vi "Temperature Limit.vi"() -> ()   [LabVIEW 2012]
doc: "该VI可仿真温度采集，绘制温度图形，并通知用户温度是否超出范围。"
panel:
  in  "开始":bool
  in  "△t(ms)":i32(slide)=400 scale=50.0..500.0
  in  "停止":bool
  in  "上限":dbl=28.0 format="%.2f"
  out "温度":cluster{"Temperature":dbl, "High Limit":dbl}(graph)={"Temperature"=85.88749999999999, "High Limit"=80.0}
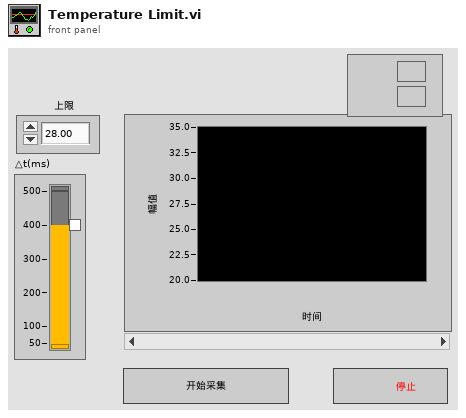
[diagram p1: front panel]
types:
  T1 = enum8{"Enabled", "Disabled", "Disabled and Grayed Out"}
  T2 = enum16{"Always On", "Always Off", "Off While Running"}
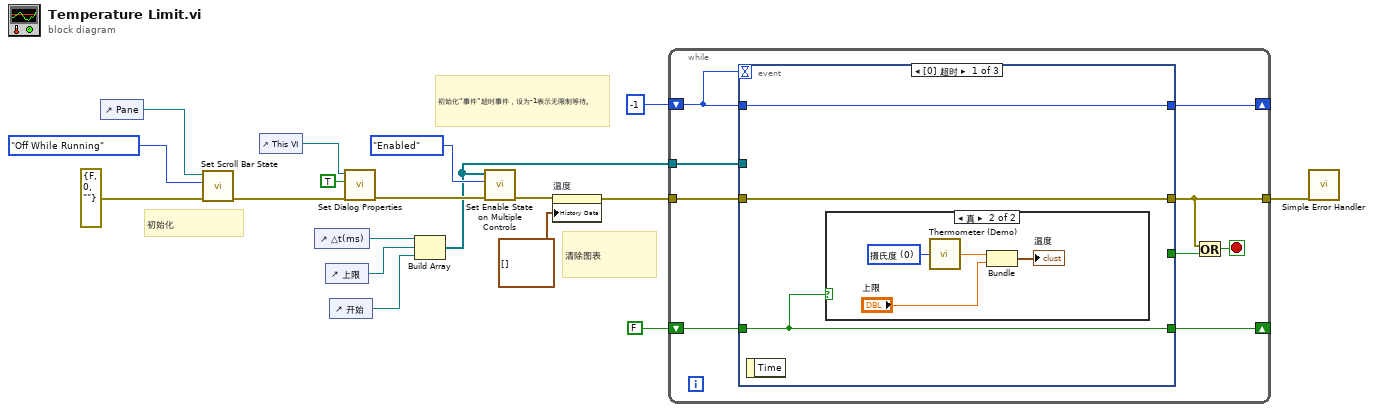
[diagram p0: block diagram]
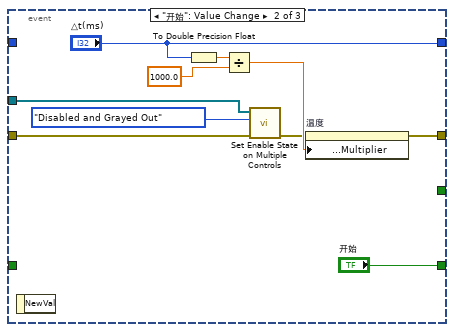
[diagram p3: hidden frame]
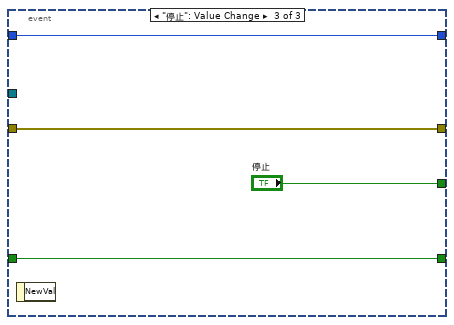
[diagram p4: hidden frame]
diagram:
  # "清除图表"
  # "初始化“事件”超时事件，设为-1表示无限制等待。"
  # "初始化"
  n1 = control-ref of="Pane"() -> (w11:refnum<vi>)
  n2 = call "Set Scroll Bar State.vi"("错误输入"=cluster{"状态":bool, "代码":i32, "源":string} {"状态"=FALSE, "代码"=0, "源"=""} ("错误输入（无错误）"), "滚动条可见（始终打开）"=T2."Off While Running", "窗格引用输入"=w11) -> ("错误输出"=w9:cluster{"状态":bool, "代码":i32, "源":string})  [unwired: 7 in, 1 out]
  n3 = control-ref of="This VI"() -> (w10:refnum<vi>)
  n4 = control-ref of="△t(ms)"() -> (w5:refnum<vi>)
  n5 = control-ref of="上限"() -> (w4:refnum<vi>)
  n6 = control-ref of="开始"() -> (w3:refnum<vi>)
  n7 = call "Set Dialog Properties.vi"("错误输入（无错误）"=w9, "启用对话框属性"=TRUE, "VI引用输入"=w10) -> ("错误输出"=w7:cluster{"状态":bool, "代码":i32, "源":string})  [unwired: 7 in, 1 out]
  n8 = Build Array ("创建数组")(w5, w4, w3) -> (w1:refnum<vi>[])
  n9 = call "Set Enable State on Multiple Controls.vi"("错误输入"=w7, "已禁用状态"=T1."Enabled", "控件"=w1) -> ("错误输出"=w6:cluster{"状态":bool, "代码":i32, "源":string})  [unwired: 8 in]
  n10 = property on="温度" class="WFChart (严格)"(error in=w6, "History Data"=cluster{"温度":dbl, "高限制":dbl}[] [] ("历史数据")) -> (error out=w17:errorcluster)  [unwired: 1 in, 1 out]
  n11 = while {
    tunnel: w17 -> [w27]
    tunnel: [w25] -> w15
    shift-right: [w23] -> _
    shift-left: FALSE ("开始") -> [w22]
    shift-right: [w21] -> _
    shift-left: -1 ("△t(ms)") -> [w20]
    tunnel: w1 -> [w19]
    stop <- w26 stop-if-true
    n12 = event shown="[0] 超时" {
      selector: _ -> [_ _ _]
      dyn-events: _ -> [_ _ _]
      timeout: w20 -> [_ _ _]
      tunnel: [_ _ "停止"] -> w24
      tunnel: w27 -> [w30 w37 w47]
      tunnel: [w30 w44 w47] -> w25
      tunnel: [w28 "开始" w46] -> w23
      tunnel: w22 -> [w28 _ w46]
      tunnel: [w29 "△t(ms)" w45] -> w21
      tunnel: w20 -> [w29 _ w45]
      tunnel: w19 -> [_ w35 _]
      event Timeout {
        n13 = event-data ("事件数据节点")() -> ()  [unwired: 1 in, 1 out]
        n14 = case shown="真" w28 {
          frame False {
          }
          frame True {
            w31 = u16 0 items=["摄氏度", "华氏度"] ("单位（0：摄氏度）")
            n15 = call "Thermometer (Demo).vi"("单位（0：摄氏度）"=w31) -> ("温度值"=w32:dbl)
            n16 = Bundle ("捆绑")("温度值"=w32, "上限"="上限") -> (→"温度":cluster{"温度值":dbl, "上限":dbl})  [unwired: 1 in]
          }
        }
      }
      event "开始": Value Change {
        n17 = event-data ("事件数据节点")() -> ()  [unwired: 1 in, 1 out]
        n18 = To Double Precision Float ("转换为双精度浮点数")(number="△t(ms)") -> (double precision float=w43:dbl)
        n19 = Divide ("除")(x=w43, y=1000.0) -> (x/y=w41:dbl)
        n20 = call "Set Enable State on Multiple Controls.vi"("错误输入"=w37, "已禁用状态"=T1."Disabled and Grayed Out", "控件"=w35) -> ("错误输出"=w36:cluster{"状态":bool, "代码":i32, "源":string})  [unwired: 8 in]
        n21 = property on="温度" class="WFChart (严格)"(error in=w36, "X Scale.Offset and Multiplier:Multiplier"=w41) -> (error out=w44:errorcluster)  [unwired: 1 in, 1 out]
      }
      event "停止": Value Change {
        n22 = event-data ("事件数据节点")() -> ()  [unwired: 1 in, 1 out]
      }
    }
    n23 = Or ("或")(x=w25, y=w24) -> (x .or. y?=w26:bool)
  }
  n24 = call <vilib>:"Simple Error Handler.vi"("error in (no error)"=w15) -> ()  [unwired: 4 in, 5 out]
